vi "Plugin - Long Measurement.vi"(11 "Message Queues in":T1) -> ()   [LabVIEW 2019]
uses:
  support/Copy of Message Queue/All Message Queues.ctl
  support/Copy of Message Queue/Message Cluster.ctl
  support/Message Queue/Message Queue.lvlib
  support/Copy of Message Queue/Copy of Message Queue.lvlib
panel:
  in  "Long Measurement(m)":dbl format="%.4g"
  in  "error in":errorcluster
  out "error out":errorcluster
  in  "Next":bool
  in  "Exit":bool
  # "Enter Long Measurement"
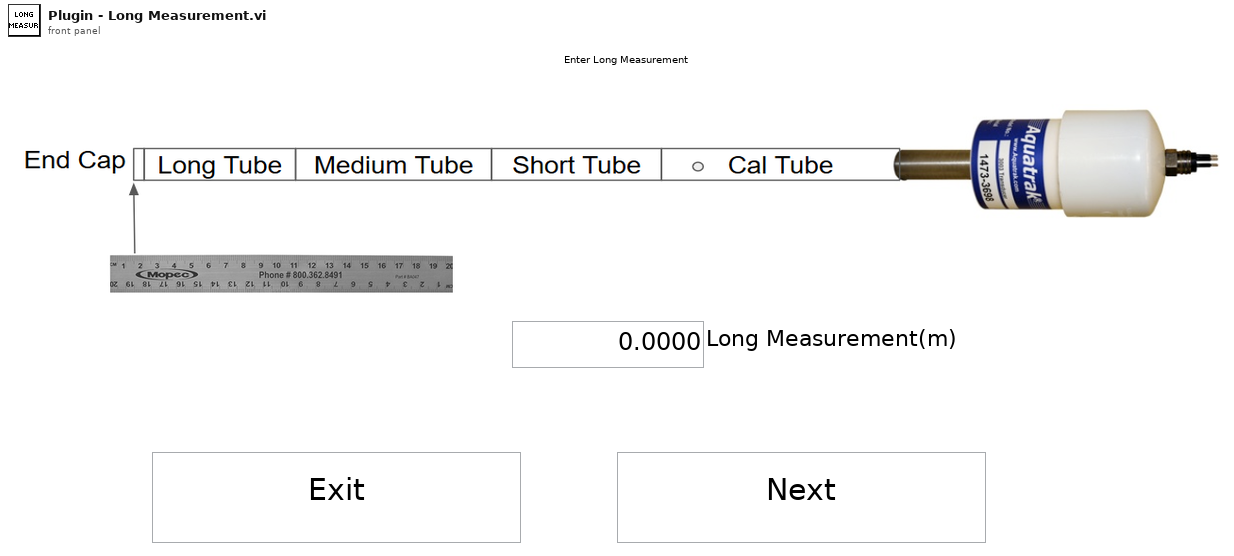
[diagram p1: front panel]
types:
  T1 = typedef "Copy of Message Queue.lvlib/All Message Queues.ctl" = cluster{"UI":refnum<queue>, "Acquisition":refnum<queue>, "Logging":refnum<queue>, "Analyze":refnum<queue>}
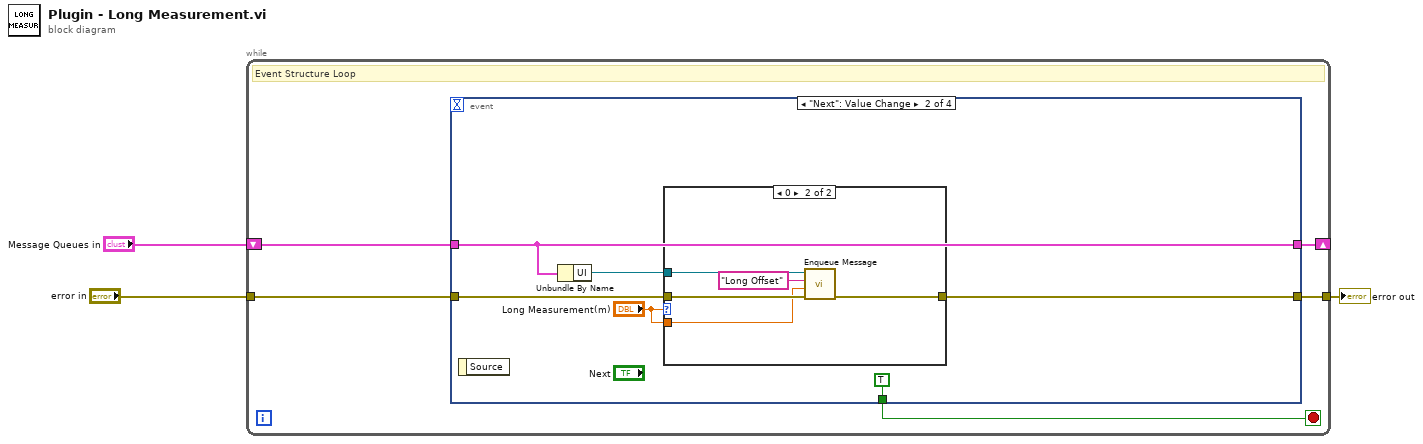
[diagram p0: block diagram]
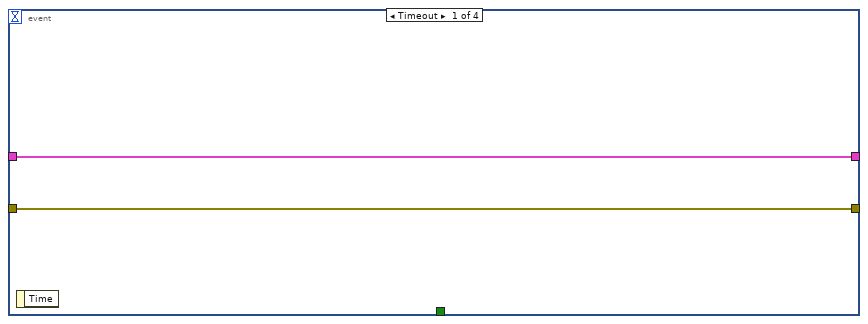
[diagram p2: hidden frame]
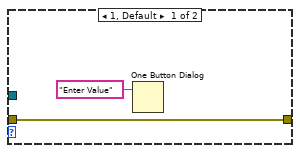
[diagram p3: hidden frame]
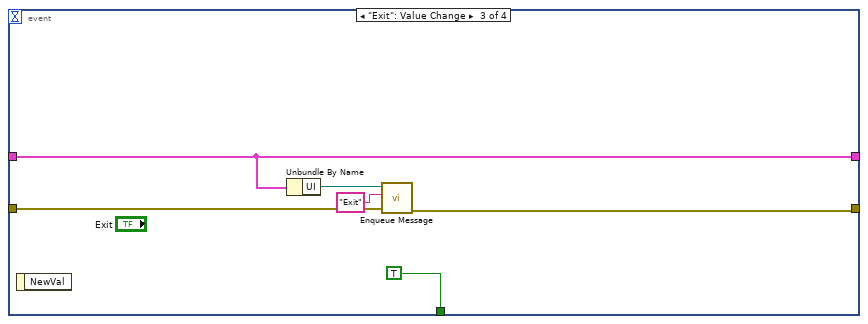
[diagram p4: hidden frame]
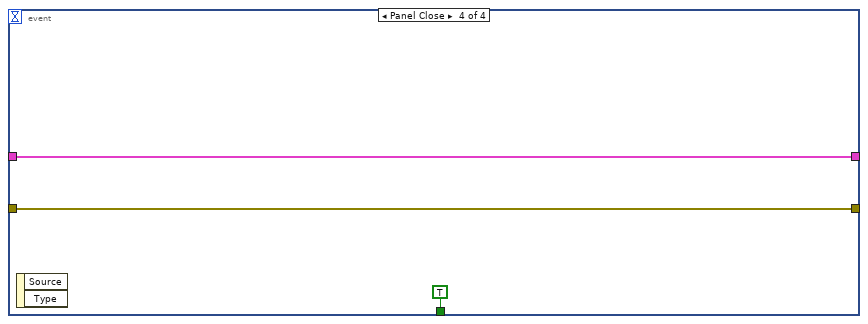
[diagram p5: hidden frame]
diagram:
  n1 = while {
    shift-right: [w7] -> _
    shift-left: "Message Queues in" -> [w6]
    tunnel: [w5] -> w2
    tunnel: "error in" -> [w4]
    stop <- w8 stop-if-true
    # "Event Structure Loop"
    n2 = event shown="[1] \"Next\": Value Change" {
      selector: _ -> [_ _ _ _]
      dyn-events: _ -> [_ _ _ _]
      timeout: _ -> [_ _ _ _]
      tunnel: [_ TRUE ("NewVal") TRUE ("NewVal") TRUE ("NewVal")] -> w8
      tunnel: w6 -> [w10 w16 w26 w32]
      tunnel: [w10 w16 w26 w32] -> w7
      tunnel: [w9 w13 w24 w30] -> w5
      tunnel: w4 -> [w9 w12 w25 w30]
      event Timeout {
        n3 = event-data() -> ()  [unwired: 1 in, 1 out]
      }
      event "Next": Value Change {
        n4 = event-data() -> ()  [unwired: 1 in, 1 out]
        n5 = Unbundle By Name(w16) -> ("UI"=w15:refnum<queue>)
        n6 = case shown="0" "Long Measurement(m)" {
          tunnel: w15 -> [_ w22]
          tunnel: [w18 w21] -> w13
          tunnel: w12 -> [w18 w20]
          tunnel: "Long Measurement(m)" -> [_ w19]
          frame 1, Default {
            n7 = One Button Dialog(message="Enter Value") -> ()  [unwired: 1 in, 1 out]
          }
          frame 0 {
            n8 = call "Enqueue Message.vi"("error in (no error)"=w20, "Message Data"=w19, "Message"="Long Offset", "Message Queue"=w22) -> ("error out"=w21:errorcluster)  [unwired: 6 in, 1 out]
          }
        }
      }
      event "Exit": Value Change {
        n9 = event-data() -> ()  [unwired: 1 in, 1 out]
        n10 = Unbundle By Name(w26) -> ("UI"=w27:refnum<queue>)
        n11 = call "Enqueue Message.vi"("error in (no error)"=w25, "Message"="Exit", "Message Queue"=w27) -> ("error out"=w24:errorcluster)  [unwired: 7 in, 1 out]
      }
      event Panel Close {
        n12 = event-data() -> ()  [unwired: 1 in, 2 out]
      }
    }
  }
  "error out" <- w2
